vi "Robot_listen.vi"(8 "error in (no error)":errorcluster, 11 "connection ID IN":refnum<k5>) -> (0 "error IO":errorcluster, 2 "robotmessage":string, 3 "connection ID OUT":refnum<k5>)   [LabVIEW 2024]
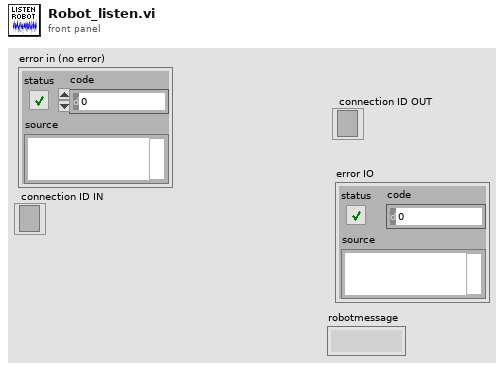
[diagram p1: front panel]
types:
  T1 = enum16{"Standard", "Buffered", "CRLF", "Immediate"}
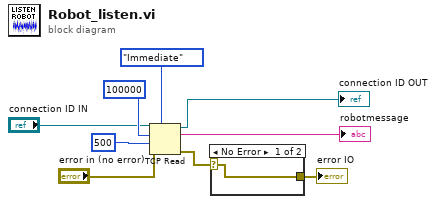
[diagram p0: block diagram]
diagram:
  n1 = TCP Read(connection ID="connection ID IN", bytes to read=100000, error in (no error)="error in (no error)", 7:T1."Immediate" ("mode (standard)"), 9:500 ("timeout ms (25000)")) -> (connection ID out=→"connection ID OUT":refnum<k5>, data out=→"robotmessage":string, error out=w7:errorcluster)
  n2 = case shown="No Error" w7 {
    selector: w7 -> [w10 _]
    tunnel: [w10 _] -> w1
    frame No Error {
    }
    frame Error {
    }
  }
  "error IO" <- w1
